vi "WFS Set Trigger Delay.vi"(8 "error in (no error)":errorcluster {"code" format="%.0x"}, 10 "Trigger Delay Set":i32 format="%.0g", 11 "instrument handle":refnum<visa-resource-name>) -> (0 "error out":errorcluster {"code" format="%.0x"}, 2 "Trigger Delay Act":i32, 3 "instrument handle out":refnum<visa-resource-name>)   [LabVIEW 2020]
doc: "This VI sets an additional trigger delay for a hardware trigger mode set by VI SetTriggerMode()."
uses:
  WFS_32.dll
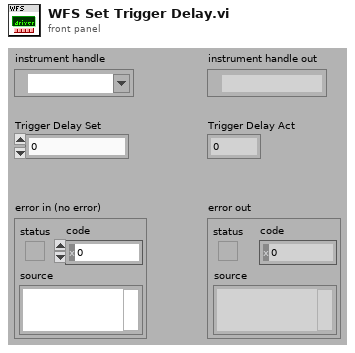
[diagram p1: front panel]
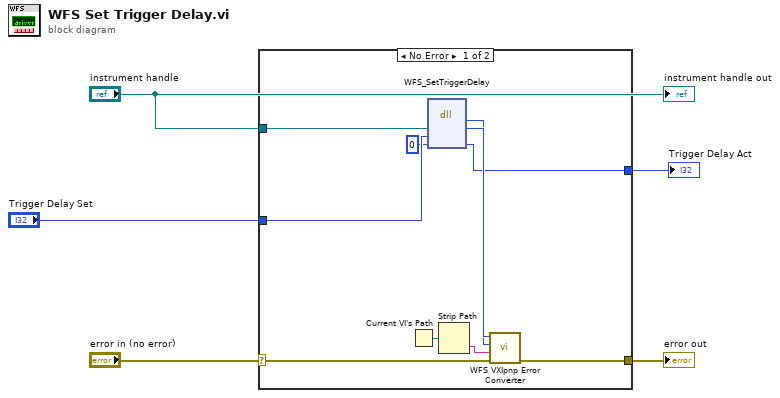
[diagram p0: block diagram]
diagram:
  n1 = case shown="No Error" "error in (no error)" {
    selector: "error in (no error)" -> [w10 w16]
    tunnel: [w9 w16] -> w5
    tunnel: "instrument handle" -> [w14 _]
    tunnel: "Trigger Delay Set" -> [w8 _]
    tunnel: [w6 _] -> w1
    frame No Error {
      n2 = Current VI's Path() -> (path=w15:path)
      n3 = dll-call lib="WFS_*.*" fn="WFS_SetTriggerDelay"("Instrument Handle"=w14, "Trigger Delay Set"=w8, "Trigger Delay Act"=0) -> (w12:i32, "Instrument Handle"=w13:u32, "Trigger Delay Act"=w6:i32)  [unwired: 4 in, 2 out]
      n4 = Strip Path(path=w15) -> (name=w11:string)  [unwired: 1 out]
      n5 = call "WFS VXIpnp Error Converter.vi"("error in (no error)"=w10, "Name Of VI (\"\")"=w11, "CVI Error Code (0)"=w12, "instrument handle"=w13) -> ("error out"=w9:errorcluster)  [unwired: 6 in, 1 out]
    }
    frame Error {
    }
  }
  "error out" <- w5
  "Trigger Delay Act" <- w1
  "instrument handle out" <- "instrument handle"
